vi "Create Connections.vi"(8 "error in (no error)":errorcluster, 11 "RT Data Cluster in":T1={"Timekeeper hdl"="", "clkDisc session"=variant, "Compiled Data"={"SyncMod?"=FALSE, "SyncMod"="", "ConnectionSettings"={"Mode"=enum."Generate sample clock", "pxitrig"=FALSE, "pfi0"=FALSE, "pfi1"=FALSE, "pfi2"=FALSE, "External Pin"=enum."PFI0", "Routes"=[], "pxitrig1_ts"=FALSE}, "TimeKeeper"="", "ScanOffset(%)"=0.0, "StartDelay(s)"=0, "Time Ref Settings"={"Time Reference"=enum."GPS", "Priority 1"=0, "Priority 2"=0, "IRIG type"=enum."IRIGB AM", "Terminal"="", "PPSSetTime"=FALSE, "Start Time"=timestamp(0 s since 1904-01-01)}, "FIFO Locations"={"SysTime"=[], "TimeRef"=[], "Status"=[]}, "Clock and Trigger Routing"={"Shared Trigger Source Terminal (Master Chassis)"="PXI_Trig0", "Master Trigger Output"="PFI0", "Export Clock"=FALSE, "Export Trigger"=FALSE}}, "OutputsData"=[], "OutputsFIFO"=refnum, "Scan Period"=0, "Timekeeper type"=enum."6683", "SyncMod type"=enum."6683", "SyncMod hdl"=""} {"Compiled Data"."Time Ref Settings"."Priority 2" min=0 max=255; "Compiled Data"."Time Ref Settings"."Priority 1" min=0 max=255}) -> (0 "error out":errorcluster, 3 "RT Data Cluster out":T1={"Timekeeper hdl"="", "clkDisc session"=variant, "Compiled Data"={"SyncMod?"=FALSE, "SyncMod"="", "ConnectionSettings"={"Mode"=enum."Generate sample clock", "pxitrig"=FALSE, "pfi0"=FALSE, "pfi1"=FALSE, "pfi2"=FALSE, "External Pin"=enum."PFI0", "Routes"=[], "pxitrig1_ts"=FALSE}, "TimeKeeper"="", "ScanOffset(%)"=0.0, "StartDelay(s)"=0, "Time Ref Settings"={"Time Reference"=enum."GPS", "Priority 1"=0, "Priority 2"=0, "IRIG type"=enum."IRIGB AM", "Terminal"="", "PPSSetTime"=FALSE, "Start Time"=timestamp(0 s since 1904-01-01)}, "FIFO Locations"={"SysTime"=[], "TimeRef"=[], "Status"=[]}, "Clock and Trigger Routing"={"Shared Trigger Source Terminal (Master Chassis)"="PXI_Trig0", "Master Trigger Output"="PFI0", "Export Clock"=FALSE, "Export Trigger"=FALSE}}, "OutputsData"=[], "OutputsFIFO"=refnum, "Scan Period"=0, "Timekeeper type"=enum."6683", "SyncMod type"=enum."6683", "SyncMod hdl"=""} {"Compiled Data"."Time Ref Settings"."Priority 2" min=0 max=255; "Compiled Data"."Time Ref Settings"."Priority 1" min=0 max=255})   [LabVIEW 2017, in "Chassis TimeSync Engine.lvlib"]
uses:
  Chassis TimeSync Engine.lvlib
  RT Data Cluster.ctl
  mdevClkDisc.llb/_clkDisc_session.ctl
  Shared/Compiled Data.ctl
  Shared/Connection Settings.ctl
  Shared/Mode.ctl
  Shared/External Pin.ctl
  Shared/Routes.ctl
  Shared/Route.ctl
  Shared/Time Ref Settings.ctl
  Shared/Time Reference.ctl
  Shared/IRIG Type.ctl
  System Explorer/ClockTrigger_routing.ctl
  timekeeper type.ctl
  Timekeeper Route Pin.ctl
  <instrlib>/niSync/niSync.llb/niSync Create Clock (Frequency).vi
  Shared/Chassis TimeSync Shared.lvlib
  System Explorer/Chassis TimeSync System Explorer.lvlib
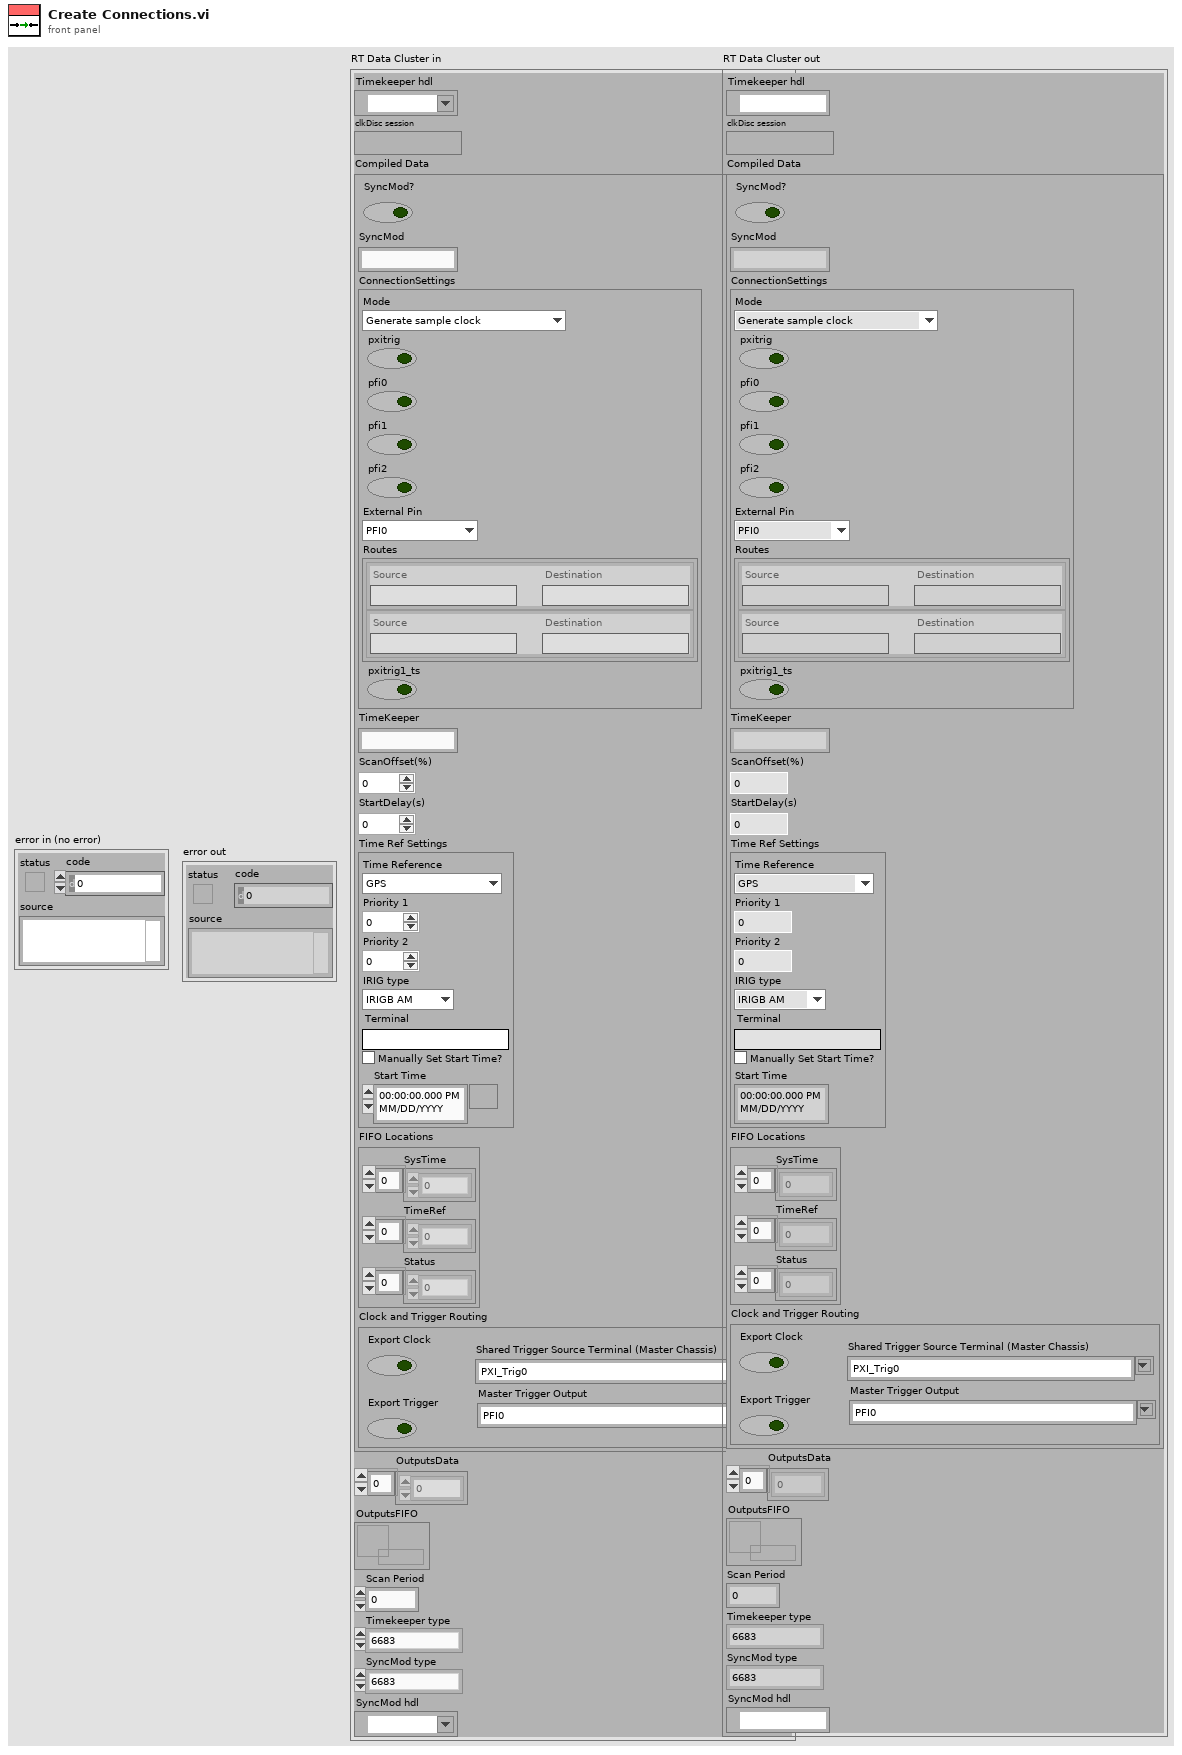
[diagram p1: front panel]
types:
  T1 = typedef "Chassis TimeSync Engine.lvlib/RT Data Cluster.ctl" = cluster{"Timekeeper hdl":refnum<k15>, "clkDisc session":T2, "Compiled Data":T3, "OutputsData":dbl[], "OutputsFIFO":refnum<k33>, "Scan Period":u32, "Timekeeper type":T13, "SyncMod type":T13, "SyncMod hdl":refnum<k15>}
  T2 = typedef "_clkDisc_session.ctl" = variant
  T3 = typedef "Chassis TimeSync Shared.lvlib/Compiled Data.ctl" = cluster{"SyncMod?":bool, "SyncMod":string, "ConnectionSettings":T4, "TimeKeeper":string, "ScanOffset(%)":dbl, "StartDelay(s)":u16, "Time Ref Settings":T9, "FIFO Locations":cluster{"SysTime":i32[], "TimeRef":i32[], "Status":i32[]}, "Clock and Trigger Routing":T12}
  T4 = typedef "Chassis TimeSync Shared.lvlib/Connection Settings.ctl" = cluster{"Mode":T5, "pxitrig":bool, "pfi0":bool, "pfi1":bool, "pfi2":bool, "External Pin":T6, "Routes":T7, "pxitrig1_ts":bool}
  T5 = typedef "Chassis TimeSync Shared.lvlib/Mode.ctl" = enum16{"Generate sample clock", "Route sample clock out of chassis", "Route sample clock into chassis", "Custom routes"}
  T6 = typedef "Chassis TimeSync Shared.lvlib/External Pin.ctl" = enum16{"PFI0", "PFI1", "PFI2"}
  T7 = typedef "Chassis TimeSync Shared.lvlib/Routes.ctl" = T8[]
  T8 = typedef "Chassis TimeSync Shared.lvlib/Route.ctl" = cluster{"Source":string, "Destination":string}
  T9 = typedef "Chassis TimeSync Shared.lvlib/Time Ref Settings.ctl" = cluster{"Time Reference":T10, "Priority 1":i32, "Priority 2":i32, "IRIG type":T11, "Terminal":string, "PPSSetTime":bool, "Start Time":timestamp}
  T10 = typedef "Chassis TimeSync Shared.lvlib/Time Reference.ctl" = enum16{"GPS", "IRIG", "PPS", "1588 Ordinary Clock", "PXI Chassis Clock", "Free Running (Internal)"}
  T11 = typedef "Chassis TimeSync Shared.lvlib/IRIG Type.ctl" = enum16{"IRIGB DC", "IRIGB AM"}
  T12 = typedef "Chassis TimeSync System Explorer.lvlib/ClockTrigger_routing.ctl" = cluster{"Shared Trigger Source Terminal (Master Chassis)":string, "Master Trigger Output":string, "Export Clock":bool, "Export Trigger":bool}
  T13 = typedef "Chassis TimeSync Engine.lvlib/timekeeper type.ctl" = enum16{"6683", "6683H", "6682", "6682H", "non-timekeeper", "timekeeper"}
  T14 = typedef "Chassis TimeSync Engine.lvlib/Timekeeper Route Pin.ctl" = enum16{"TTL0", "TTL1", "PFI0", "PFI1", "PFI2", "PXI_Clk10", "PXI_Clk10_In", "BoardClk", "ClkOut", "Oscillator"}
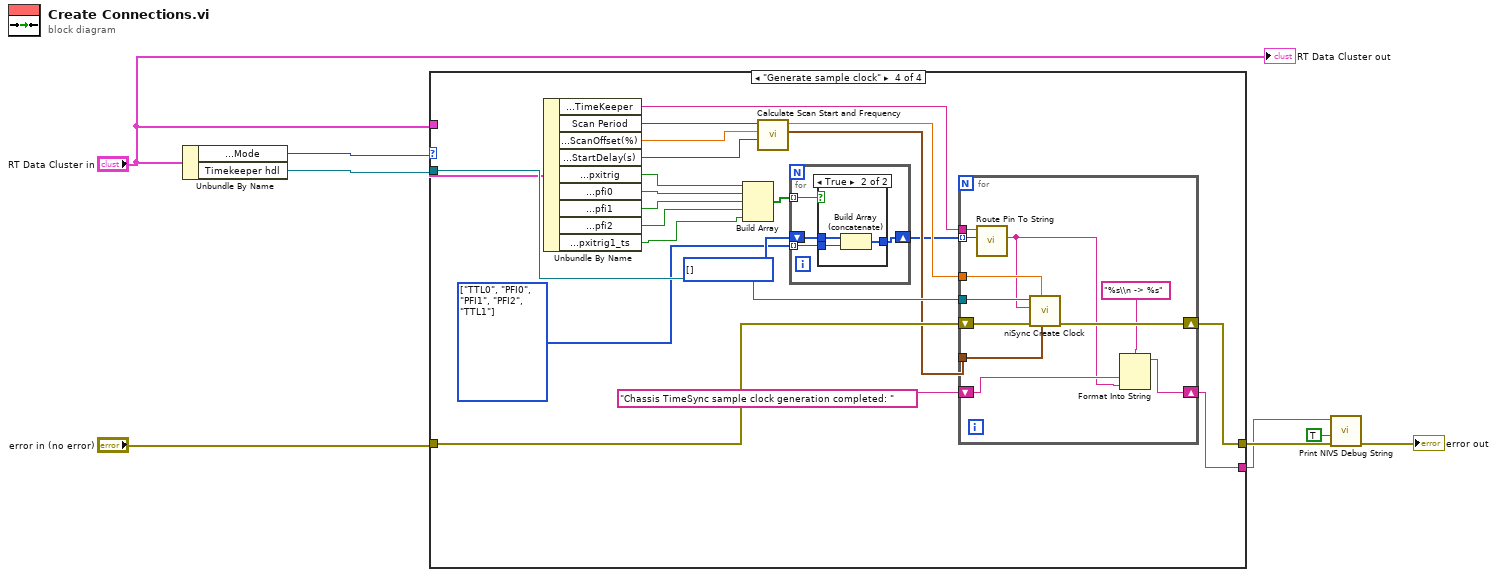
[diagram p0: block diagram]
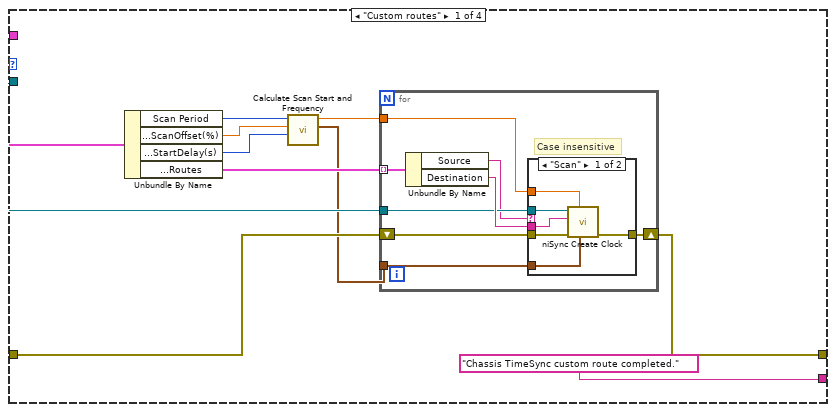
[diagram p2: hidden frame]
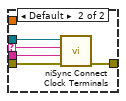
[diagram p3: hidden frame]
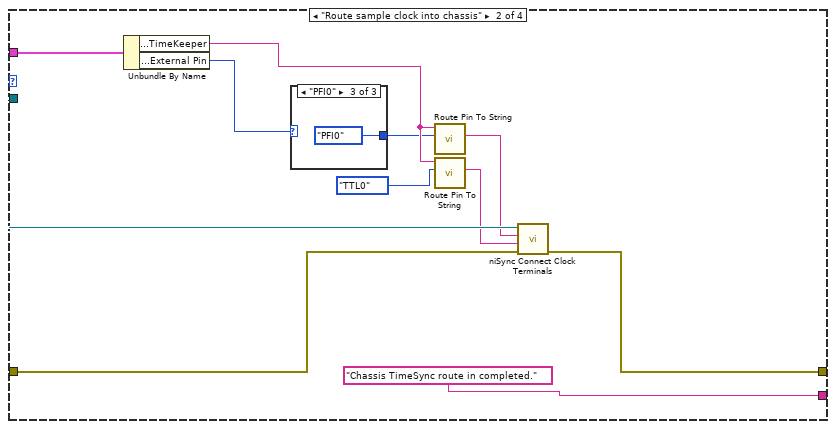
[diagram p4: hidden frame]
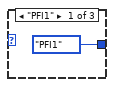
[diagram p5: hidden frame]
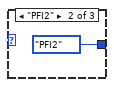
[diagram p6: hidden frame]
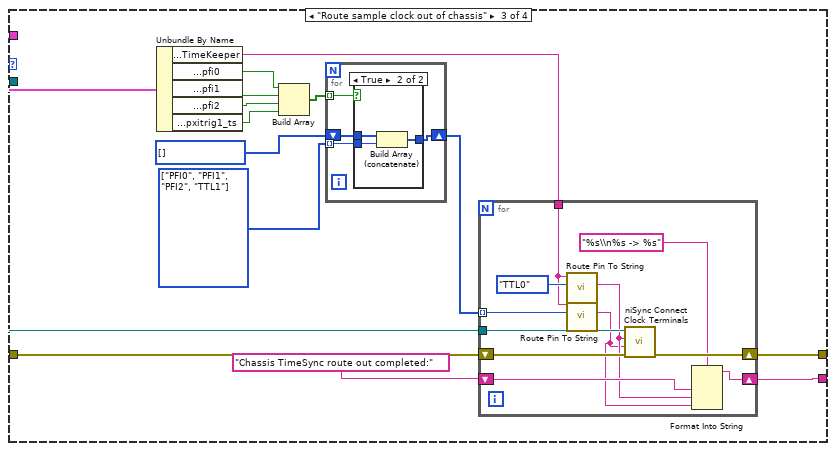
[diagram p7: hidden frame]
diagram:
  n1 = Unbundle By Name("RT Data Cluster in") -> ("Compiled Data.ConnectionSettings.Mode"=w8:T5, "Timekeeper hdl"=w7:refnum<k15>)
  n2 = case shown="\"Generate sample clock\"" w8 {
    tunnel: "error in (no error)" -> [w18 w39 w65 w105]
    tunnel: w7 -> [w14 w43 w64 w106]
    tunnel: "RT Data Cluster in" -> [w19 w49 w67 w104]
    tunnel: [w16 w47 w66 w107] -> w4
    tunnel: ["Chassis TimeSync custom route completed." "Chassis TimeSync route in completed." w53 w87] -> w2
    frame "Custom routes" {
      n3 = Unbundle By Name(w19) -> ("Scan Period"=w13:u32, "Compiled Data.ScanOffset(%)"=w12:dbl, "Compiled Data.StartDelay(s)"=w11:u16, "Compiled Data.ConnectionSettings.Routes"=w17:T7)
      n4 = call "Calculate Scan Start and Frequency.vi"("Start delay (s)"=w11, "Start offset (fraction)"=w12, "Scan Period (uS)"=w13) -> ("Start time"=w9:timestamp, "Frequency"=w10:dbl)  [unwired: 7 in]
      n5 = for {
        shift-right: [w24] -> w16
        shift-left: w18 -> [w27]
        tunnel: w17 -> [w26] mode=indexing
        tunnel: w14 -> [w23]
        tunnel: w10 -> [w21]
        tunnel: w9 -> [w20]
        # "Case insensitive"
        n6 = Unbundle By Name(w26) -> ("Source"=w22:string, "Destination"=w25:string)
        n7 = case shown="\"Scan\"" w22 {
          selector: w22 -> [_ w34]
          tunnel: w27 -> [w33 w38]
          tunnel: w25 -> [w28 w37]
          tunnel: [w32 w36] -> w24
          tunnel: w23 -> [w31 w35]
          tunnel: w21 -> [w30 _]
          tunnel: w20 -> [w29 _]
          frame "Scan" {
            n8 = call-poly <instrlib>:"niSync Create Clock.vi"("start time"=w29, "frequency"=w30, "error in (no error)"=w33, "terminal"=w28, "instrument handle"=w31) -> ("error out"=w32:errorcluster)  [unwired: 3 in, 3 out]
          }
          frame Default {
            n9 = call <instrlib>:"niSync Connect Clock Terminals.vi"("error in (no error)"=w38, "destination terminal"=w37, "source terminal"=w34, "instrument handle"=w35) -> ("error out"=w36:errorcluster)  [unwired: 6 in, 1 out]
          }
        }
      }
    }
    frame "Route sample clock into chassis" {
      n10 = Unbundle By Name(w49) -> ("Compiled Data.TimeKeeper"=w46:string, "Compiled Data.ConnectionSettings.External Pin"=w48:T6)
      n11 = case shown="\"PFI0\"" w48 {
        tunnel: [Timekeeper_Route_Pin."PFI1" ("Pin") Timekeeper_Route_Pin."PFI2" ("Pin") Timekeeper_Route_Pin."PFI0" ("Pin")] -> w44
        frame "PFI1" {
        }
        frame "PFI2" {
        }
        frame "PFI0" {
        }
      }
      n12 = call "Route Pin To String.vi"("Pin"=w44, "Module"=w46) -> ("String"=w42:string)  [unwired: 9 in]
      n13 = call "Route Pin To String.vi"("Pin"=Timekeeper_Route_Pin."TTL0", "Module"=w46) -> ("String"=w41:string)  [unwired: 9 in]
      n14 = call <instrlib>:"niSync Connect Clock Terminals.vi"("error in (no error)"=w39, "destination terminal"=w41, "source terminal"=w42, "instrument handle"=w43) -> ("error out"=w47:errorcluster)  [unwired: 6 in, 1 out]
    }
    frame "Route sample clock out of chassis" {
      w57 = T14[] [enum."PFI0", enum."PFI1", enum."PFI2", enum."TTL1"] items=["TTL0", "TTL1", "PFI0", "PFI1", "PFI2", "PXI_Clk10", "PXI_Clk10_In", "BoardClk", "ClkOut", "Oscillator"]
      w58 = T14[] [] items=["TTL0", "TTL1", "PFI0", "PFI1", "PFI2", "PXI_Clk10", "PXI_Clk10_In", "BoardClk", "ClkOut", "Oscillator"]
      n15 = Unbundle By Name(w67) -> ("Compiled Data.TimeKeeper"=w63:string, "Compiled Data.ConnectionSettings.pfi0"=w62:bool, "Compiled Data.ConnectionSettings.pfi1"=w61:bool, "Compiled Data.ConnectionSettings.pfi2"=w60:bool, "Compiled Data.ConnectionSettings.pxitrig1_ts"=w55:bool)
      n16 = Build Array(w62, w61, w60, w55) -> (w59:bool[])
      n17 = for {
        tunnel: w59 -> [w71] mode=indexing
        shift-right: [w68] -> w56
        shift-left: w58 -> [w70]
        tunnel: w57 -> [w69] mode=indexing
        n18 = case shown="True" w71 {
          tunnel: w70 -> [w72 w75]
          tunnel: w69 -> [_ w74]
          tunnel: [w72 w73] -> w68
          frame False {
          }
          frame True {
            n19 = Build Array (concatenate)(w75, w74) -> (w73:T14[])
          }
        }
      }
      n20 = for {
        tunnel: w64 -> [w84]
        shift-right: [w86] -> w66
        shift-left: w65 -> [w85]
        tunnel: w63 -> [w82]
        tunnel: w56 -> [w81] mode=indexing
        shift-right: [w77] -> w53
        shift-left: "Chassis TimeSync route out completed:" -> [w80]
        n21 = call "Route Pin To String.vi"("Pin"=Timekeeper_Route_Pin."TTL0", "Module"=w82) -> ("String"=w79:string)  [unwired: 9 in]
        n22 = call "Route Pin To String.vi"("Pin"=w81, "Module"=w82) -> ("String"=w78:string)  [unwired: 9 in]
        n23 = call <instrlib>:"niSync Connect Clock Terminals.vi"("error in (no error)"=w85, "destination terminal"=w78, "source terminal"=w79, "instrument handle"=w84) -> ("error out"=w86:errorcluster)  [unwired: 6 in, 1 out]
        n24 = Format Into String(format string="%s\\n%s -> %s", w80, w79, w78) -> (resulting string=w77:string)  [unwired: 2 in, 1 out]
      }
    }
    frame "Generate sample clock" {
      w96 = T14[] [enum."TTL0", enum."PFI0", enum."PFI1", enum."PFI2", enum."TTL1"] items=["TTL0", "TTL1", "PFI0", "PFI1", "PFI2", "PXI_Clk10", "PXI_Clk10_In", "BoardClk", "ClkOut", "Oscillator"]
      w97 = T14[] [] items=["TTL0", "TTL1", "PFI0", "PFI1", "PFI2", "PXI_Clk10", "PXI_Clk10_In", "BoardClk", "ClkOut", "Oscillator"]
      n25 = Unbundle By Name(w104) -> ("Compiled Data.TimeKeeper"=w94:string, "Scan Period"=w103:u32, "Compiled Data.ScanOffset(%)"=w102:dbl, "Compiled Data.StartDelay(s)"=w101:u16, "Compiled Data.ConnectionSettings.pxitrig"=w93:bool, "Compiled Data.ConnectionSettings.pfi0"=w92:bool, "Compiled Data.ConnectionSettings.pfi1"=w91:bool, "Compiled Data.ConnectionSettings.pfi2"=w90:bool, "Compiled Data.ConnectionSettings.pxitrig1_ts"=w89:bool)
      n26 = Build Array(w93, w92, w91, w90, w89) -> (w98:bool[])
      n27 = call "Calculate Scan Start and Frequency.vi"("Start delay (s)"=w101, "Start offset (fraction)"=w102, "Scan Period (uS)"=w103) -> ("Start time"=w99:timestamp, "Frequency"=w100:dbl)  [unwired: 7 in]
      n28 = for {
        tunnel: w98 -> [w111] mode=indexing
        shift-right: [w108] -> w95
        shift-left: w97 -> [w110]
        tunnel: w96 -> [w109] mode=indexing
        n29 = case shown="True" w111 {
          tunnel: w110 -> [w112 w115]
          tunnel: w109 -> [_ w114]
          tunnel: [w112 w113] -> w108
          frame False {
          }
          frame True {
            n30 = Build Array (concatenate)(w115, w114) -> (w113:T14[])
          }
        }
      }
      n31 = for {
        shift-right: [w125] -> w107
        shift-left: w105 -> [w126]
        tunnel: w106 -> [w124]
        tunnel: w100 -> [w123]
        tunnel: w99 -> [w122]
        tunnel: w95 -> [w121] mode=indexing
        tunnel: w94 -> [w120]
        shift-right: [w118] -> w87
        shift-left: "Chassis TimeSync sample clock generation completed: " -> [w117]
        n32 = call "Route Pin To String.vi"("Pin"=w121, "Module"=w120) -> ("String"=w116:string)  [unwired: 9 in]
        n33 = call-poly <instrlib>:"niSync Create Clock.vi"("start time"=w122, "frequency"=w123, "error in (no error)"=w126, "terminal"=w116, "instrument handle"=w124) -> ("error out"=w125:errorcluster)  [unwired: 3 in, 3 out]
        n34 = Format Into String(format string="%s\\n -> %s", w117, w116) -> (resulting string=w118:string)  [unwired: 2 in, 1 out]
      }
    }
  }
  n35 = call "Print NIVS Debug String.vi"("error in (no error)"=w4, "Add to NIVS Log FIle? (T)"=TRUE, "Debug String"=w2) -> ("error out"=→"error out":errorcluster)  [unwired: 7 in]
  "RT Data Cluster out" <- "RT Data Cluster in"
